vi "ReadGFGandWriteALLtoINI.vi"(8 "error in (no error)":errorcluster, 11 "Path":path) -> (0 "error out":errorcluster)   [LabVIEW 2012]
doc: "This VI reads an INI file and stores all keys in a Generalized Functional Global Variable (GFG). It then monitors updates to the GFG and writes keys back into INI file before closing. Note that the INI file only supports data type DBL or STRING. The GFG can handle any arbitrary data type, but values that are not DBL or STRING are discarded when closing and not written to INI file."
uses:
  <vilib>/Utility/config.llb/Write Key (Double).vi
  <vilib>/Utility/config.llb/Write Key (String).vi
  <vilib>/Utility/config.llb/Write Key (Boolean).vi
  <vilib>/Utility/config.llb/NI_LVConfig.lvlib
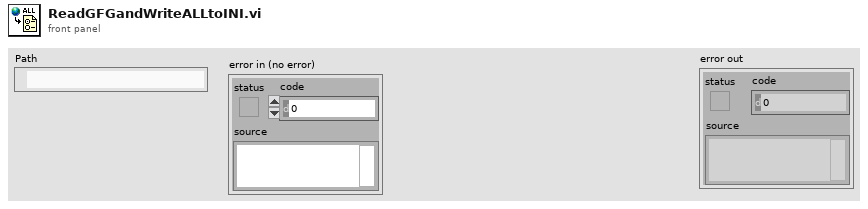
[diagram p1: front panel]
types:
  T1 = typedef "NI_LVConfig.lvlib/Config Data RefNum.ctl" = refnum<k1>
  T2 = typedef "VariantType.lvlib/Type.ctl" = enum8{"Invalid Type", "Void", "I8", "I16", "I32", "I64", "U8", "U16", "U32", "U64", "Single Float", "Double Float", "Extended Float", "Single Complex", "Double Complex", "Extended Complex", "Enum U8", "Enum U16", "Enum U32", "Enum U64", "Single Float With Unit", "Double Float With Unit", "Extended Float With Unit", "Single Complex with Unit", "Double Complex with Unit", "Extended Complex with Unit", "Boolean", "String", "Path", "Picture", "Tag", "Array", "Cluster", "Variant", "LV Variant", "Waveform", "Timestamp", "Digital Waveform", "Digital Data", "ExpressData", "Refnum", "External Data", "VI", "Poly VI", "LabVIEW Class Instance", "Fixed Point"}
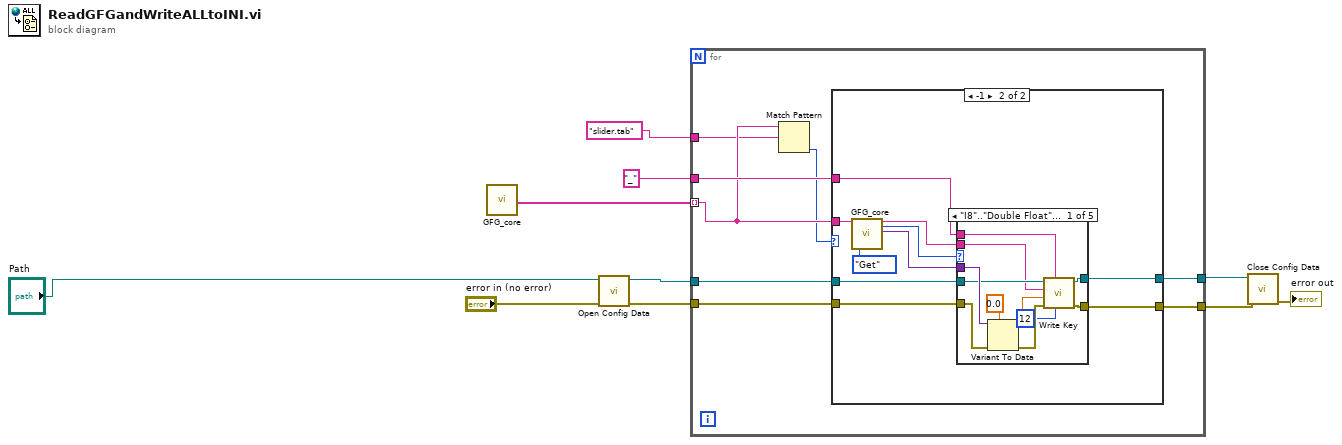
[diagram p0: block diagram]
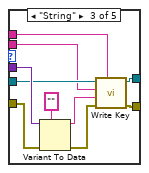
[diagram p4: hidden frame]
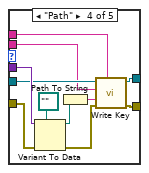
[diagram p5: hidden frame]
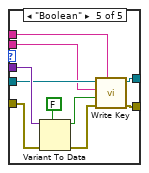
[diagram p6: hidden frame]
diagram:
  n1 = call "GFG_core.vi"() -> ("All Variable Names Out"=w3:string[])  [unwired: 13 in, 6 out]
  n2 = call <vilib>:"Open Config Data.vi"("error in (no error)"="error in (no error)", "configuration file path"="Path") -> ("error out"=w8:errorcluster, "refnum"=w9:T1)  [unwired: 7 in, 1 out]
  n3 = for {
    tunnel: [w17] -> w5
    tunnel: w9 -> [w16]
    tunnel: w8 -> [w18]
    tunnel: [w15] -> w6
    tunnel: w3 -> [w13] mode=indexing
    tunnel: "_" ("Variable Name") -> [w14]
    tunnel: "slider.tab" ("regular expression") -> [w12]
    n4 = Match Pattern(string=w13, regular expression=w12) -> (offset past match=w11:i32)  [unwired: 1 in, 3 out]
    n5 = case shown="-1" w11 {
      tunnel: w18 -> [w19 w27]
      tunnel: [w19 w26] -> w17
      tunnel: w16 -> [w20 w25]
      tunnel: [w20 w24] -> w15
      tunnel: w14 -> [_ w22]
      tunnel: w13 -> [_ w21]
      frame 0, Default {
      }
      frame -1 {
        n6 = call "GFG_core.vi"("Variable Name in"=w21, "Action"=enum16{"Init", "Set", "Get"}."Get") -> ("Variable Name Out"=w23:string, "Data Type Out"=w29:T2, "Variant Out"=w28:variant)  [unwired: 11 in, 4 out]
        n7 = case shown="\"I8\"..\"Double Float\", \"Enum U8\"..\"Enum U64\"" w29 {
          tunnel: w28 -> [w40 _ w53 w64 w74]
          tunnel: [w37 w43 w50 w62 w71] -> w26
          tunnel: w27 -> [w36 w43 w49 w61 w70]
          tunnel: w25 -> [w35 w42 w48 w60 w69]
          tunnel: [w34 w42 w47 w59 w68] -> w24
          tunnel: w23 -> [w33 _ w46 w58 w67]
          tunnel: w22 -> [w32 _ w45 w57 w66]
          frame "I8".."Double Float", "Enum U8".."Enum U64" {
            n8 = Variant To Data(error in=w36, type=0.0, Variant=w40) -> (data=w39:dbl, error out=w38:errorcluster)
            n9 = call-poly <vilib>:"Write Key.vi"("precision (6)"=i16 12, "section"=w32, "error in (no error)"=w38, "value"=w39, "key"=w33, "refnum"=w35) -> ("error out"=w37:errorcluster, "refnum out"=w34:T1)  [unwired: 3 in, 1 out]
          }
          frame Default {
          }
          frame "String" {
            n10 = Variant To Data(error in=w49, type="" ("Variable Name Out"), Variant=w53) -> (data=w52:string, error out=w51:errorcluster)
            n11 = call-poly <vilib>:"Write Key.vi"("section"=w45, "error in (no error)"=w51, "value"=w52, "key"=w46, "refnum"=w48) -> ("error out"=w50:errorcluster, "refnum out"=w47:T1)  [unwired: 4 in, 1 out]
          }
          frame "Path" {
            n12 = Variant To Data(error in=w61, type=path "" ("configuration file path 2"), Variant=w64) -> (data=w54:path, error out=w63:errorcluster)
            n13 = Path To String(path=w54) -> (string=w55:string)
            n14 = call-poly <vilib>:"Write Key.vi"("section"=w57, "error in (no error)"=w63, "value"=w55, "key"=w58, "refnum"=w60) -> ("error out"=w62:errorcluster, "refnum out"=w59:T1)  [unwired: 4 in, 1 out]
          }
          frame "Boolean" {
            n15 = Variant To Data(error in=w70, type=FALSE, Variant=w74) -> (data=w73:bool, error out=w72:errorcluster)
            n16 = call-poly <vilib>:"Write Key.vi"("section"=w66, "error in (no error)"=w72, "value"=w73, "key"=w67, "refnum"=w69) -> ("error out"=w71:errorcluster, "refnum out"=w68:T1)  [unwired: 4 in, 1 out]
          }
        }
      }
    }
  }
  n17 = call <vilib>:"Close Config Data.vi"("error in (no error)"=w5, "refnum"=w6) -> ("error out"=→"error out":errorcluster)  [unwired: 8 in, 1 out]
